vi "Graph Get Y scale Settings.vi"(8 "error in (no error)":errorcluster, 10 "Active Y Scale":i32, 11 "Chart Ref":refnum<vi>) -> (0 "error out":errorcluster, 1 "Y scale":T1)   [LabVIEW 2011]
uses:
  Y scale cluster.ctl
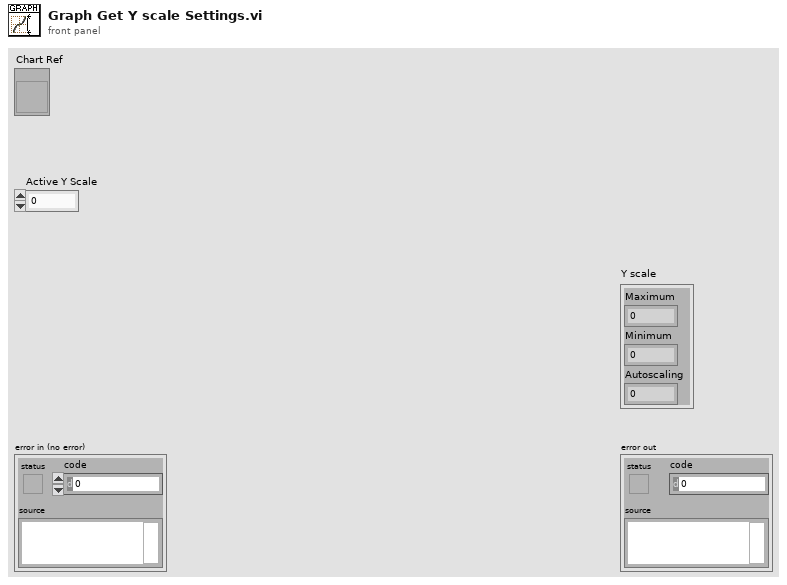
[diagram p1: front panel]
types:
  T1 = typedef "Y scale cluster.ctl" = cluster{"Maximum":dbl, "Minimum":dbl, "Autoscaling":i32}
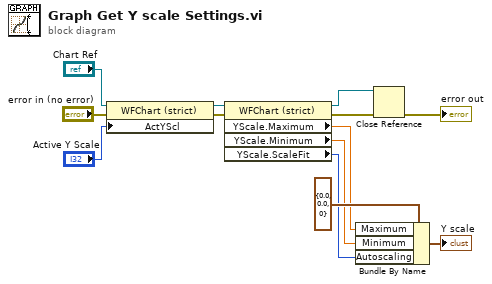
[diagram p0: block diagram]
diagram:
  n1 = property class="WFChart (strict)"(reference="Chart Ref", error in="error in (no error)", "ActYScl"="Active Y Scale") -> (reference out=w13:refnum<vi>, error out=w12:errorcluster)
  n2 = property class="WFChart (strict)"(reference=w13, error in=w12) -> (reference out=w8:refnum<vi>, error out=w7:errorcluster, "YScale.Maximum"=w4:dbl, "YScale.Minimum"=w3:dbl, "YScale.ScaleFit"=w2:u8)
  n3 = Bundle By Name(cluster=T1 {"Maximum"=0.0, "Minimum"=0.0, "Autoscaling"=0} ("Y scale"), "Maximum"=w4, "Minimum"=w3, "Autoscaling"=w2) -> (→"Y scale":T1)
  n4 = Close Reference(reference=w8, error in (no error)=w7) -> (error out=→"error out":errorcluster)
